vi "Func-엑셀 데이터를 그래프로 출력.vi"() -> ()   [LabVIEW 2015] (continued)
2.46\t3.252\n3.3\t2.47\t3.256\n3.3\t2.48\t3.262\n3.3\t2.49\t3.268\n3.3\t2.5\t3.273\n3.3\t2.51\t3.277\n3.3\t2.51\t3.284\n3.3\t2.52\t3.298\n3.3\t2.52\t3.307\n3.3\t2.52\t3.316\n3.3\t2.53\t3.327\n3.3\t2.54\t3.339\n3.3\t2.55\t3.347\n3.3\t2.56\t3.356\n3.3\t2.57\t3.363\n3.3\t2.57\t3.367\n3.3\t2.58\t3.375\n3.3\t2.59\t3.377\n3.3\t2.6\t3.382\n3.3\t2.6\t3.39\n3.3\t2.61\t3.395\n3.3\t2.61\t3.399\n3.3\t2.62\t3.409\n3.3\t2.63\t3.418\n3.3\t2.63\t3.427\n3.3\t2.64\t3.434\n3.3\t2.65\t3.441\n3.3\t2.66\t3.45\n3.3\t2.66\t3.465\n3.3\t2.67\t3.473\n3.3\t2.68\t3.483\n3.3\t2.68\t3.494\n3.3\t2.69\t3.499\n3.3\t2.69\t3.509\n3.3\t2.69\t3.51\n3.3\t2.7\t3.515\n3.3\t2.71\t3.521\n3.3\t2.72\t3.524\n3.3\t2.72\t3.532\n3.3\t2.73\t3.539\n3.3\t2.73\t3.546\n3.3\t2.74\t3.551\n3.3\t2.74\t3.562\n3.3\t2.75\t3.568\n3.3\t2.75\t3.574\n3.3\t2.76\t3.581\n3.3\t2.77\t3.592\n3.3\t2.78\t3.6\n3.3\t2.78\t3.607\n3.3\t2.78\t3.611\n3.3\t2.79\t3.618\n3.3\t2.79\t3.63\n3.3\t2.8\t3.637\n3.3\t2.81\t3.639\n3.3\t2.81\t3.649\n3.3\t2.82\t3.659\n3.3\t2.83\t3.666\n3.3\t2.83\t3.673\n3.3\t2.84\t3.677\n3.3\t2.84\t3.684\n3.3\t2.85\t3.693\n3.3\t2.86\t3.697\n3.3\t2.86\t3.702\n3.3\t2.86\t3.708\n3.3\t2.86\t3.714\n3.3\t2.87\t3.724\n3.3\t2.87\t3.732\n3.3\t2.88\t3.736\n3.3\t2.89\t3.743\n3.3\t2.9\t3.753\n3.3\t2.9\t3.761\n3.3\t2.91\t3.766\n3.3\t2.91\t3.775\n3.3\t2.92\t3.788\n3.3\t2.92\t3.795\n3.3\t2.93\t3.804\n3.3\t2.93\t3.813\n3.3\t2.94\t3.823\n3.3\t2.94\t3.83\n3.3\t2.94\t3.834\n3.3\t2.95\t3.841\n3.3\t2.95\t3.85\n3.3\t2.96\t3.857\n3.3\t2.96\t3.86\n3.3\t2.97\t3.871\n3.3\t2.97\t3.877\n3.3\t2.98\t3.883\n3.3\t2.98\t3.893\n3.3\t2.99\t3.893\n3.3\t2.99\t3.9\n3.3\t3\t3.911\n3.3\t3\t3.917\n3.3\t3.01\t3.923\n3.3\t3.01\t3.93\n3.3\t3.02\t3.941\n3.3\t3.03\t3.946\n3.3\t3.03\t3.955\n3.3\t3.03\t3.96\n3.3\t3.03\t3.966\n3.3\t3.04\t3.977\n3.3\t3.04\t3.982\n3.3\t3.05\t3.99\n3.3\t3.05\t3.994\n3.3\t3.06\t4.004\n3.3\t3.06\t4.013\n3.3\t3.07\t4.021\n3.3\t3.07\t4.027\n3.3\t3.08\t4.036\n3.3\t3.08\t4.048\n3.3\t3.08\t4.053\n3.3\t3.09\t4.055\n3.3\t3.09\t4.064\n3.3\t3.1\t4.072\n3.3\t3.1\t4.076\n3.3\t3.11\t4.085\n3.3\t3.11\t4.09\n3.3\t3.11\t4.101\n3.3\t3.11\t4.107\n3.3\t3.11\t4.112\n3.3\t3.11\t4.122\n3.3\t3.12\t4.13\n3.3\t3.13\t4.139\n3.3\t3.13\t4.146\n3.3\t3.13\t4.16\n3.3\t3.13\t4.169\n3.3\t3.14\t4.169\n3.3\t3.14\t4.18\n3.3\t3.14\t4.187\n3.3\t3.15\t4.194\n3.3\t3.15\t4.197\n3.3\t3.16\t4.204\n3.3\t3.16\t4.214\n3.3\t3.16\t4.223\n3.3\t3.17\t4.23\n3.3\t3.17\t4.24\n3.3\t3.18\t4.248\n3.3\t3.18\t4.254\n3.3\t3.19\t4.258\n3.3\t3.19\t4.264\n3.3\t3.2\t4.266\n3.3\t3.2\t4.275\n3.3\t3.2\t4.28\n3.3\t3.2\t4.286\n3.3\t3.2\t4.298\n3.3\t3.21\t4.309\n3.3\t3.21\t4.317\n3.3\t3.21\t4.324\n3.3\t3.21\t4.329\n3.3\t3.22\t4.336\n3.3\t3.22\t4.342\n3.3\t3.22\t4.346\n3.3\t3.23\t4.354\n3.3\t3.23\t4.366\n3.3\t3.23\t4.375\n3.3\t3.24\t4.381\n3.3\t3.25\t4.391\n3.3\t3.25\t4.398\n3.3\t3.25\t4.406\n3.3\t3.26\t4.41\n3.3\t3.26\t4.415\n3.3\t3.26\t4.424\n3.3\t3.26\t4.436\n3.3\t3.26\t4.44\n3.3\t3.27\t4.445\n3.3\t3.27\t4.453\n3.3\t3.27\t4.461\n3.3\t3.28\t4.468\n3.3\t3.28\t4.476\n3.3\t3.28\t4.484\n3.3\t3.28\t4.489\n3.3\t3.28\t4.502\n3.3\t3.28\t4.507\n3.3\t3.29\t4.512\n3.3\t3.29\t4.519\n3.3\t3.3\t4.527\n3.3\t3.3\t4.533\n3.3\t3.3\t4.542\n3.3\t3.3\t4.55\n3.3\t3.3\t4.555\n3.3\t3.31\t4.562\n3.3\t3.31\t4.566\n3.3\t3.31\t4.575\n3.3\t3.31\t4.582\n3.3\t3.32\t4.591\n3.3\t3.32\t4.597\n3.3\t3.32\t4.608\n3.3\t3.33\t4.616\n3.3\t3.33\t4.62\n3.3\t3.33\t4.629\n3.3\t3.33\t4.632\n3.3\t3.33\t4.641\n3.3\t3.33\t4.646\n3.3\t3.34\t4.649\n3.3\t3.34\t4.658\n3.3\t3.34\t4.668\n3.3\t3.35\t4.68\n3.3\t3.35\t4.686\n3.3\t3.35\t4.7\n3.3\t3.35\t4.709\n3.3\t3.35\t4.714\n3.3\t3.35\t4.721\n3.3\t3.36\t4.727\n3.3\t3.36\t4.732\n3.3\t3.36\t4.739\n3.3\t3.37\t4.746\n3.3\t3.37\t4.753\n3.3\t3.37\t4.764\n3.3\t3.37\t4.769\n3.3\t3.37\t4.774\n3.3\t3.37\t4.78\n3.3\t3.37\t4.786\n3.3\t3.37\t4.791\n3.3\t3.37\t4.8\n3.3\t3.37\t4.805\n3.3\t3.37\t4.813\n3.3\t3.37\t4.82\n3.3\t3.38\t4.827\n3.3\t3.38\t4.836\n3.3\t3.38\t4.843\n3.3\t3.39\t4.846\n3.3\t3.39\t4.853\n3.3\t3.39\t4.863\n3.3\t3.39\t4.873\n3.3\t3.38\t4.88\n3.3\t3.39\t4.887\n3.3\t3.39\t4.898\n3.3\t3.39\t4.902\n3.3\t3.4\t4.912\n3.3\t3.4\t4.915\n3.3\t3.4\t4.919\n3.3\t3.4\t4.929\n3.3\t3.41\t4.936\n3.3\t3.41\t4.945\n3.3\t3.41\t4.953\n3.3\t3.41\t4.96\n3.3\t3.41\t4.966\n3.3\t3.41\t4.976\n3.3\t3.41\t4.98\n3.3\t3.41\t4.984\n3.3\t3.41\t4.991\n3.3\t3.41\t4.996\n3.3\t3.42\t5.005\n3.3\t3.41\t5.016\n3.3\t3.4\t5.02\n3.3\t3.39\t5.027\n3.3\t3.38\t5.039\n3.3\t3.37\t5.047\n3.3\t3.36\t5.052\n3.3\t3.35\t5.058\n3.3\t3.34\t5.068\n3.3\t3.33\t5.078\n3.3\t3.32\t5.085\n3.3\t3.31\t5.091\n3.3\t3.3\t5.096\n3.3\t3.33\t5.103\n3.3\t3.33\t5.109\n3.3\t3.33\t5.115\n3.3\t3.33\t5.127\n3.3\t3.33\t5.135\n3.3\t3.33\t5.145\n3.3\t3.33\t5.152\n3.3\t3.33\t5.162\n3.3\t3.33\t5.167\n3.3\t3.33\t5.174\n3.3\t3.33\t5.179\n3.3\t3.33\t5.183\n3.3\t3.33\t5.193\n3.3\t3.33\t5.2\n3.3\t3.33\t5.207\n3.3\t3.33\t5.214\n3.3\t3.33\t5.217\n3.3\t3.33\t5.229\n3.3\t3.33\t5.236\n3.3\t3.33\t5.238\n3.3\t3.33\t5.247\n3.3\t3.33\t5.259\n3.3\t3.33\t5.268\n3.3\t3.33\t5.275\n3.3\t3.33\t5.282\n3.3\t3.33\t5.289\n3.3\t3.33\t5.295\n3.3\t3.33\t5.3\n3.3\t3.33\t5.305\n3.3\t3.33\t5.311\n3.3\t3.33\t5.321\n3.3\t3.33\t5.329\n3.3\t3.33\t5.339\n3.3\t3.33\t5.343\n3.3\t3.33\t5.353\n3.3\t3.33\t5.363\n3.3\t3.33\t5.368\n3.3\t3.33\t5.375\n3.3\t3.33\t5.382\n3.3\t3.33\t5.388\n3.3\t3.33\t5.391\n3.3\t3.33\t5.396\n3.3\t3.33\t5.407\n3.3\t3.33\t5.409\n3.3\t3.33\t5.418\n3.3\t3.33\t5.426\n3.3\t3.33\t5.436\n3.3\t3.33\t5.441\n3.3\t3.33\t5.447\n3.3\t3.33\t5.455\n3.3\t3.33\t5.459\n3.3\t3.33\t5.467\n3.3\t3.33\t5.469\n3.3\t3.33\t5.478\n3.3\t3.33\t5.487\n3.3\t3.33\t5.495\n3.3\t3.33\t5.5\n3.3\t3.33\t5.507\n3.3\t3.33\t5.516\n3.3\t3.33\t5.525\n3.3\t3.33\t5.531\n3.3\t3.33\t5.536\n3.3\t3.33\t5.547\n3.3\t3.33\t5.553\n3.3\t3.33\t5.557\n3.3\t3.33\t5.561\n3.3\t3.33\t5.568\n3.3\t3.33\t5.574\n3.3\t3.33\t5.58\n3.3\t3.33\t5.589\n3.3\t3.33\t5.596\n3.3\t3.33\t5.605\n3.3\t3.33\t5.609\n3.3\t3.33\t5.617\n3.3\t3.33\t5.629\n3.3\t3.33\t5.634\n3.3\t3.33\t5.642\n3.3\t3.33\t5.654\n3.3\t3.33\t5.661\n3.3\t3.33\t5.666\n3.3\t3.33\t5.672\n3.3\t3.33\t5.678\n3.3\t3.33\t5.684\n3.3\t3.33\t5.692\n3.3\t3.33\t5.696\n3.3\t3.33\t5.704\n3.3\t3.33\t5.711\n3.3\t3.33\t5.721\n3.3\t3.33\t5.725\n3.3\t3.33\t5.737\n3.3\t3.33\t5.745\n3.3\t3.33\t5.752\n3.3\t3.33\t5.758\n3.3\t3.33\t5.761\n3.3\t3.33\t5.767\n3.3\t3.33\t5.776\n3.3\t3.33\t5.782\n3.3\t3.33\t5.789\n3.3\t3.33\t5.802\n3.3\t3.33\t5.809\n3.3\t3.33\t5.816\n3.3\t3.33\t5.816\n3.3\t3.33\t5.822\n3.3\t3.33\t5.826\n3.3\t3.33\t5.832\n3.3\t3.33\t5.839\n3.3\t3.33\t5.843\n3.3\t3.33\t5.859\n3.3\t3.33\t5.866\n3.3\t3.33\t5.873\n3.3\t3.33\t5.885\n3.3\t3.33\t5.89\n3.3\t3.33\t5.9\n3.3\t3.33\t5.907\n3.3\t3.33\t5.913\n3.3\t3.33\t5.916\n3.3\t3.33\t5.923\n3.3\t3.33\t5.927\n3.3\t3.33\t5.932\n3.3\t3.33\t5.939\n3.3\t3.33\t5.945\n3.3\t3.33\t5.953\n3.3\t3.33\t5.963\n3.3\t3.33\t5.971\n3.3\t3.33\t5.975\n3.3\t3.33\t5.984\n3.3\t3.33\t5.991\n3.3\t3.33\t5.998\n3.3\t3.33\t6.007\n3.3\t3.33\t6.012\n3.3\t3.33\t6.02\n3.3\t3.33\t6.026\n3.3\t3.33\t6.029\n3.3\t3.33\t6.036\n3.3\t3.33\t6.038\n3.3\t3.33\t6.046\n3.3\t3.33\t6.052\n3.3\t3.33\t6.063\n3.3\t3.33\t6.07\n3.3\t3.33\t6.076\n3.3\t3.33\t6.084\n3.3\t3.33\t6.087\n3.3\t3.33\t6.092\n3.3\t3.33\t6.099\n3.3\t3.33\t6.104\n3.3\t3.33\t6.108\n3.3\t3.33\t6.118\n3.3\t3.33\t6.128\n3.3\t3.33\t6.137\n3.3\t3.33\t6.144\n3.3\t3.33\t6.153\n3.3\t3.33\t6.161\n3.3\t3.33\t6.169\n3.3\t3.33\t6.175\n3.3\t3.33\t6.18\n3.3\t3.33\t6.187\n3.3\t3.33\t6.189\n3.3\t3.33\t6.195\n3.3\t3.33\t6.203\n3.3\t3.33\t6.207\n3.3\t3.33\t6.213\n3.3\t3.33\t6.222\n3.3\t3.33\t6.229\n3.3\t3.33\t6.239\n3.3\t3.33\t6.242\n3.3\t3.33\t6.248\n3.3\t3.33\t6.258\n3.3\t3.33\t6.264\n3.3\t3.33\t6.27\n3.3\t3.33\t6.277\n3.3\t3.33\t6.286\n3.3\t3.33\t6.288\n3.3\t3.33\t6.289\n3.3\t3.33\t6.297\n3.3\t3.33\t6.303\n3.3\t3.33\t6.311\n3.3\t3.33\t6.318\n3.3\t3.33\t6.327\n3.3\t3.33\t6.34\n3.3\t3.33\t6.342\n3.3\t3.33\t6.348\n3.3\t3.33\t6.356\n3.3\t3.33\t6.363\n3.3\t3.33\t6.37\n3.3\t3.33\t6.374\n3.3\t3.33\t6.382\n3.3\t3.33\t6.388\n3.3\t3.33\t6.392\n3.3\t3.33\t6.394\n3.3\t3.33\t6.401\n3.3\t3.33\t6.407\n3.3\t3.33\t6.412\n3.3\t3.33\t6.42\n3.3\t3.33\t6.431\n3.3\t3.33\t6.439\n3.3\t3.33\t6.445\n3.3\t3.33\t6.452\n3.3\t3.33\t6.456\n3.3\t3.33\t6.463\n3.3\t3.33\t6.47\n3.3\t3.33\t6.475\n3.3\t3.33\t6.48\n3.3\t3.33\t6.491\n3.3\t3.33\t6.497\n3.3\t3.33\t6.499\n3.3\t3.33\t6.509\n3.3\t3.33\t6.512\n3.3\t3.33\t6.518\n3.3\t3.33\t6.527\n3.3\t3.33\t6.534\n3.3\t3.33\t6.544\n3.3\t3.33\t6.548\n3.3\t3.33\t6.555\n3.3\t3.33\t6.563\n3.3\t3.33\t6.57\n3.3\t3.33\t6.572\n3.3\t3.33\t6.577\n3.3\t3.33\t6.586\n3.3\t3.33\t6.591\n3.3\t3.33\t6.597\n3.3\t3.33\t6.607\n3.3\t3.33\t6.616\n3.3\t3.33\t6.622\n3.3\t3.33\t6.632\n3.3\t3.32\t6.638\n3.3\t3.32\t6.638\n3.3\t3.32\t6.643\n3.3\t3.32\t6.646\n3.3\t3.32\t6.65\n3.3\t3.32\t6.656\n3.3\t3.32\t6.66\n3.3\t3.32\t6.668\n3.3\t3.32\t6.675\n3.3\t3.32\t6.682\n3.3\t3.32\t6.69\n3.3\t3.32\t6.699\n3.3\t3.32\t6.706\n3.3\t3.32\t6.709\n3.3\t3.32\t6.718\n3.3\t3.32\t6.723\n3.3\t3.32\t6.728\n3.3\t3.32\t6.738\n3.3\t3.32\t6.747\n3.3\t3.32\t6.756\n3.3\t3.32\t6.765\n3.3\t3.32\t6.773\n3.3\t3.32\t6.778\n3.3\t3.32\t6.781\n3.3\t3.32\t6.784\n3.3\t3.32\t6.786\n3.3\t3.32\t6.793\n3.3\t3.32\t6.797\n3.3\t3.32\t6.802\n3.3\t3.32\t6.807\n3.3\t3.32\t6.812\n3.3\t3.32\t6.821\n3.3\t3.32\t6.832\n3.3\t3.32\t6.837\n3.3\t3.32\t6.846\n3.3\t3.32\t6.857\n3.3\t3.32\t6.861\n3.3\t3.32\t6.866\n3.3\t3.32\t6.875\n3.3\t3.32\t6.88\n3.3\t3.32\t6.886\n3.3\t3.32\t6.893\n3.3\t3.32\t6.898\n3.3\t3.32\t6.905\n3.3\t3.32\t6.906\n3.3\t3.32\t6.913\n3.3\t3.32\t6.915\n3.3\t3.32\t6.92\n3.3\t3.32\t6.929\n3.3\t3.32\t6.933\n3.3\t3.32\t6.938\n3.3\t3.32\t6.94\n3.3\t3.32\t6.95\n3.3\t3.32\t6.959\n3.3\t3.32\t6.965\n3.3\t3.32\t6.971\n3.3\t3.32\t6.982\n3.3\t3.32\t6.992\n3.3\t3.32\t6.996\n3.3\t3.32\t7.008\n3.3\t3.31\t7.012\n3.3\t3.31\t7.018\n3.3\t3.31\t7.028\n3.3\t3.31\t7.03\n3.3\t3.31\t7.034\n3.3\t3.31\t7.037\n3.3\t3.31\t7.043\n3.3\t3.31\t7.048\n3.3\t3.31\t7.054\n3.3\t3.31\t7.061\n3.3\t3.31\t7.069\n3.3\t3.31\t7.077\n3.3\t3.31\t7.082\n3.3\t3.31\t7.088\n3.3\t3.31\t7.095\n3.3\t3.31\t7.099\n3.3\t3.31\t7.103\n3.3\t3.31\t7.109\n3.3\t3.31\t7.115\n3.3\t3.31\t7.119\n3.3\t3.31\t7.125\n3.3\t3.31\t7.131\n3.3\t3.31\t7.138\n3.3\t3.31\t7.148\n3.3\t3.31\t7.149\n3.3\t3.31\t7.158\n3.3\t3.31\t7.161\n3.3\t3.31\t7.166\n3.3\t3.31\t7.173\n3.3\t3.31\t7.177\n3.3\t3.31\t7.185\n3.3\t3.31\t7.193\n3.3\t3.31\t7.198\n3.3\t3.31\t7.202\n3.3\t3.31\t7.204\n3.3\t3.31\t7.21\n3.3\t3.31\t7.216\n3.3\t3.31\t7.22\n3.3\t3.31\t7.227\n3.3\t3.31\t7.234\n3.3\t3.31\t7.245\n3.3\t3.31\t7.25\n3.3\t3.31\t7.256\n3.3\t3.31\t7.264\n3.3\t3.31\t7.27\n3.3\t3.31\t7.273\n3.3\t3.31\t7.277\n3.3\t3.31\t7.283\n3.3\t3.31\t7.287\n3.3\t3.31\t7.293\n3.3\t3.31\t7.297\n3.3\t3.31\t7.303\n3.3\t3.31\t7.312\n3.3\t3.31\t7.317\n3.3\t3.31\t7.325\n3.3\t3.31\t7.336\n3.3\t3.31\t7.343\n3.3\t3.31\t7.349\n3.3\t3.31\t7.354\n3.3\t3.31\t7.358\n3.3\t3.31\t7.358\n3.3\t3.31\t7.362\n3.3\t3.31\t7.37\n3.3\t3.31\t7.372\n3.3\t3.31\t7.377\n3.3\t3.31\t7.383\n3.3\t3.31\t7.393\n3.3\t3.31\t7.4\n3.3\t3.31\t7.401\n3.3\t3.31\t7.41\n3.3\t3.31\t7.423\n3.3\t3.31\t7.426\n3.3\t3.31\t7.43\n3.3\t3.31\t7.434\n3.3\t3.31\t7.443\n3.3\t3.31\t7.447\n3.3\t3.31\t7.452\n3.3\t3.31\t7.458\n3.3\t3.31\t7.463\n3.3\t3.3\t7.475\n3.3\t3.31\t7.476\n3.3\t3.31\t7.48\n3.3\t3.31\t7.485\n3.3\t3.31\t7.493\n3.3\t3.31\t7.497\n3.3\t3.31\t7.503\n3.3\t3.31\t7.511\n3.3\t3.31\t7.517\n3.3\t3.31\t7.529\n3.3\t3.31\t7.534\n3.3\t3.3\t7.537\n3.3\t3.3\t7.545\n3.3\t3.3\t7.549\n3.3\t3.3\t7.553\n3.3\t3.3\t7.557\n3.3\t3.3\t7.561\n3.3\t3.3\t7.569\n3.3\t3.3\t7.579\n3.3\t3.3\t7.582\n3.3\t3.3\t7.587\n3.3\t3.3\t7.592\n3.3\t3.3\t7.597\n3.3\t3.3\t7.604\n3.3\t3.3\t7.607\n3.3\t3.3\t7.611\n3.3\t3.31\t7.616\n3.3\t3.31\t7.621\n3.3\t3.31\t7.627\n3.3\t3.31\t7.625\n3.3\t3.31\t7.63\n3.3\t3.31\t7.636\n3.3\t3.31\t7.639\n3.3\t3.31\t7.648\n3.3\t3.31\t7.648\n3.3\t3.31\t7.658\n3.3\t3.31\t7.665\n3.3\t3.31\t7.67\n3.3\t3.31\t7.678\n3.3\t3.31\t7.687\n3.3\t3.31\t7.694\n3.3\t3.31\t7.693\n3.3\t3.31\t7.702\n3.3\t3.31\t7.706\n3.3\t3.31\t7.711\n3.3\t3.31\t7.714\n3.3\t3.31\t7.72\n3.3\t3.31\t7.728\n3.3\t3.31\t7.73\n3.3\t3.31\t7.739\n3.3\t3.31\t7.742\n3.3\t3.31\t7.748\n3.3\t3.31\t7.752\n3.3\t3.31\t7.758\n3.3\t3.31\t7.767\n3.3\t3.31\t7.769\n3.3\t3.31\t7.776\n3.3\t3.31\t7.782\n3.3\t3.31\t7.789\n3.3\t3.31\t7.793\n3.3\t3.31\t7.796\n3.3\t3.31\t7.801\n3.3\t3.31\t7.807\n3.3\t3.31\t7.81\n3.3\t3.31\t7.815\n3.3\t3.31\t7.818\n3.3\t3.31\t7.827\n3.3\t3.31\t7.832\n3.3\t3.31\t7.836\n3.3\t3.31\t7.843\n3.3\t3.31\t7.847\n3.3\t3.31\t7.853\n3.3\t3.31\t7.86\n3.3\t3.3\t7.866\n3.3\t3.3\t7.871\n3.3\t3.3\t7.879\n3.3\t3.31\t7.885\n3.3\t3.31\t7.892\n3.3\t3.31\t7.898\n3.3\t3.31\t7.905\n3.3\t3.31\t7.911\n3.3\t3.31\t7.913\n3.3\t3.3\t7.917\n3.3\t3.3\t7.921\n3.3\t3.3\t7.928\n3.3\t3.3\t7.929\n3.3\t3.3\t7.93\n3.3\t3.3\t7.938\n3.3\t3.3\t7.941\n3.3\t3.3\t7.948\n3.3\t3.3\t7.952\n3.3\t3.3\t7.959\n3.3\t3.3\t7.971\n3.3\t3.3\t7.976\n3.3\t3.3\t7.982\n3.3\t3.3\t7.984\n3.3\t3.3\t7.987\n3.3\t3.3\t7.988\n3.3\t3.3\t7.993\n3.3\t3.3\t7.995\n3.3\t3.3\t8\n3.3\t3.3\t8.008\n3.3\t3.3\t8.014\n3.3\t3.3\t8.018\n3.3\t3.3\t8.023\n3.3\t3.3\t8.026\n3.3\t3.3\t8.026\n3.3\t3.3\t8.033\n3.3\t3.3\t8.036\n3.3\t3.3\t8.043\n3.3\t3.3\t8.049\n3.3\t3.3\t8.055\n3.3\t3.3\t8.064\n3.3\t3.3\t8.066\n3.3\t3.3\t8.073\n3.3\t3.3\t8.079\n3.3\t3.3\t8.087\n3.3\t3.3\t8.094\n3.3\t3.3\t8.099\n3.3\t3.3\t8.108\n3.3\t3.3\t8.111\n3.3\t3.3\t8.112\n3.3\t3.3\t8.117\n3.3\t3.3\t8.122\n3.3\t3.3\t8.123\n3.3\t3.3\t8.128\n3.3\t3.3\t8.13\n3.3\t3.3\t8.137\n3.3\t3.3\t8.141\n3.3\t3.3\t8.141\n3.3\t3.3\t8.148\n3.3\t3.3\t8.157\n3.3\t3.3\t8.162\n3.3\t3.3\t8.168\n3.3\t3.3\t8.177\n3.3\t3.3\t8.185\n3.3\t3.3\t8.19\n3.3\t3.3\t8.192\n3.3\t3.3\t8.195\n3.3\t3.3\t8.203\n3.3\t3.3\t8.208\n3.3\t3.3\t8.211\n3.3\t3.3\t8.22\n3.3\t3.3\t8.222\n3.3\t3.3\t8.232\n3.3\t3.3\t8.236\n3.3\t3.3\t8.238\n3.3\t3.3\t8.242\n3.3\t3.3\t8.248\n3.3\t3.3\t8.253\n3.3\t3.3\t8.254\n3.3\t3.3\t8.261\n3.3\t3.3\t8.265\n3.3\t3.3\t8.272\n3.3\t3.3\t8.276\n3.3\t3.3\t8.281\n3.3\t3.3\t8.287\n3.3\t3.3\t8.292\n3.3\t3.3\t8.297\n3.3\t3.3\t8.3\n3.3\t3.3\t8.305\n3.3\t3.3\t8.31\n3.3\t3.3\t8.315\n3.3\t3.3\t8.322\n3.3\t3.3\t8.326\n3.3\t3.3\t8.331\n3.3\t3.3\t8.336\n3.3\t3.3\t8.343\n3.3\t3.3\t8.346\n3.3\t3.3\t8.35\n3.3\t3.3\t8.353\n3.3\t3.3\t8.355\n3.3\t3.3\t8.364\n3.3\t3.3\t8.364\n3.3\t3.3\t8.367\n3.3\t3.3\t8.377\n3.3\t3.3\t8.384\n3.3\t3.3\t8.393\n3.3\t3.3\t8.393\n3.3\t3.3\t8.396\n3.3\t3.3\t8.4\n3.3\t3.3\t8.403\n3.3\t3.3\t8.406\n3.3\t3.3\t8.407\n3.3\t3.3\t8.413\n3.3\t3.3\t8.422\n3.3\t3.3\t8.428\n3.3\t3.3\t8.43\n3.3\t3.3\t8.434\n3.3\t3.3\t8.442\n3.3\t3.3\t8.447\n3.3\t3.3\t8.45\n3.3\t3.3\t8.454\n3.3\t3.3\t8.457\n3.3\t3.3\t8.464\n3.3\t3.3\t8.473\n3.3\t3.3\t8.475\n3.3\t3.3\t8.479\n3.3\t3.3\t8.484\n3.3\t3.3\t8.488\n3.3\t3.3\t8.489\n3.3\t3.3\t8.489\n3.3\t3.3\t8.491\n3.3\t3.3\t8.496\n3.3\t3.3\t8.504\n3.3\t3.3\t8.509\n3.3\t3.3\t8.513\n3.3\t3.3\t8.523\n3.3\t3.3\t8.529\n3.3\t3.3\t8.531\n3.3\t3.3\t8.533\n3.3\t3.3\t8.538\n3.3\t3.3\t8.54\n3.3\t3.3\t8.546\n3.3\t3.3\t8.548\n3.3\t3.3\t8.554\n3.3\t3.3\t8.562\n3.3\t3.3\t8.568\n3.3\t3.3\t8.575\n3.3\t3.3\t8.579\n3.3\t3.3\t8.584\n3.3\t3.3\t8.592\n3.3\t3.3\t8.596\n3.3\t3.3\t8.601\n3.3\t3.3\t8.603\n3.3\t3.3\t8.607\n3.3\t3.3\t8.613\n3.3\t3.3\t8.611\n3.3\t3.3\t8.617\n3.3\t3.3\t8.62\n3.3\t3.3\t8.625\n3.3\t3.3\t8.63\n3.3\t3.3\t8.632\n3.3\t3.3\t8.637\n3.3\t3.3\t8.643\n3.3\t3.3\t8.645\n3.3\t3.3\t8.651\n3.3\t3.3\t8.656\n3.3\t3.3\t8.661\n3.3\t3.3\t8.667\n3.3\t3.3\t8.672\n3.3\t3.3\t8.676\n3.3\t3.3\t8.681\n3.3\t3.3\t8.684\n3.3\t3.3\t8.688\n3.3\t3.3\t8.691\n3.3\t3.3\t8.695\n3.3\t3.3\t8.698\n3.3\t3.3\t8.705\n3.3\t3.3\t8.711\n3.3\t3.3\t8.714\n3.3\t3.3\t8.721\n3.3\t3.3\t8.726\n3.3\t3.3\t8.729\n3.3\t3.3\t8.733\n3.3\t3.3\t8.738\n3.3\t3.3\t8.739\n3.3\t3.3\t8.739\n3.3\t3.3\t8.745\n3.3\t3.3\t8.75\n3.3\t3.3\t8.754\n3.3\t3.3\t8.758\n3.3\t3.3\t8.766\n3.3\t3.3\t8.777\n3.3\t3.3\t8.779\n3.3\t3.3\t8.78\n3.3\t3.3\t8.785\n3.3\t3.3\t8.786\n3.3\t3.3\t8.792\n3.3\t3.3\t8.797\n3.3\t3.3\t8.8\n3.3\t3.3\t8.809\n3.3\t3.3\t8.817\n3.3\t3.3\t8.824\n3.3\t3.3\t8.824\n3.3\t3.3\t8.828\n3.3\t3.3\t8.834\n3.3\t3.3\t8.836\n3.3\t3.3\t8.841\n3.3\t3.3\t8.848\n3.3\t3.3\t8.853\n3.3\t3.3\t8.856\n3.3\t3.3\t8.858\n3.3\t3.3\t8.856\n3.3\t3.3\t8.863\n3.3\t3.3\t8.861\n3.3\t3.3\t8.863\n3.3\t3.3\t8.87\n3.3\t3.3\t8.873\n3.3\t3.3\t8.881\n3.3\t3.3\t8.885\n3.3\t3.3\t8.889\n3.3\t3.3\t8.895\n3.3\t3.3\t8.896\n3.3\t3.3\t8.904\n3.3\t3.3\t8.908\n3.3\t3.3\t8.911\n3.3\t3.3\t8.916\n3.3\t3.3\t8.92\n3.3\t3.3\t8.925\n3.3\t3.3\t8.928\n3.3\t3.3\t8.935\n3.3\t3.3\t8.941\n3.3\t3.3\t8.942\n3.3\t3.3\t8.944\n3.3\t3.3\t8.95\n3.3\t3.3\t8.953\n3.3\t3.3\t8.956\n3.3\t3.3\t8.959\n3.3\t3.3\t8.966\n3.3\t3.3\t8.97\n3.3\t3.3\t8.973\n3.3\t3.3\t8.98\n3.3\t3.3\t8.986\n3.3\t3.3\t8.989\n3.3\t3.3\t8.992\n3.3\t3.3\t8.999\n3.3\t3.3\t9.003\n3.3\t3.3\t9.005\n3.3\t3.3\t9.006\n3.3\t3.3\t9.014\n3.3\t3.3\t9.018\n3.3\t3.3\t9.025\n3.3\t3.3\t9.025\n3.3\t3.3\t9.028\n3.3\t3.3\t9.032\n3.3\t3.3\t9.035\n3.3\t3.3\t9.037\n3.3\t3.3\t9.043\n3.3\t3.3\t9.049\n3.3\t3.3\t9.052\n3.3\t3.3\t9.06\n3.3\t3.3\t9.062\n3.3\t3.3\t9.07\n3.3\t3.3\t9.072\n3.3\t3.3\t9.074\n3.3\t3.3\t9.077\n3.3\t3.3\t9.082\n3.3\t3.3\t9.085\n3.3\t3.3\t9.082\n3.3\t3.3\t9.089\n3.3\t3.3\t9.095\n3.3\t3.3\t9.101\n3.3\t3.3\t9.103\n3.3\t3.3\t9.105\n3.3\t3.3\t9.112\n3.3\t3.3\t9.115\n3.3\t3.3\t9.118\n3.3\t3.3\t9.116\n3.3\t3.3\t9.123\n3.3\t3.3\t9.129\n3.3\t3.3\t9.13\n3.3\t3.3\t9.134\n3.3\t3.3\t9.14\n3.3\t3.3\t9.148\n3.3\t3.3\t9.151\n3.3\t3.3\t9.151\n3.3\t3.3\t9.156\n3.3\t3.3\t9.16\n3.3\t3.3\t9.159\n3.3\t3.3\t9.161\n3.3\t3.3\t9.165\n3.3\t3.3\t9.172\n3.3\t3.3\t9.18\n3.3\t3.3\t9.186\n3.3\t3.3\t9.193\n3.3\t3.3\t9.198\n3.3\t3.3\t9.201\n3.3\t3.3\t9.202\n3.3\t3.3\t9.204\n3.3\t3.3\t9.206\n3.3\t3.3\t9.208\n3.3\t3.3\t9.212\n3.3\t3.3\t9.214\n3.3\t3.3\t9.218\n3.3\t3.3\t9.226\n3.3\t3.3\t9.229\n3.3\t3.3\t9.232\n3.3\t3.3\t9.237\n3.3\t3.3\t9.238\n3.3\t3.3\t9.239\n3.3\t3.3\t9.239\n3.3\t3.3\t9.242\n3.3\t3.3\t9.246\n3.3\t3.3\t9.251\n3.3\t3.3\t9.259\n3.3\t3.3\t9.268\n3.3\t3.3\t9.276\n3.3\t3.3\t9.279\n3.3\t3.3\t9.284\n3.3\t3.3\t9.285\n3.3\t3.3\t9.287\n3.3\t3.3\t9.288\n3.3\t3.3\t9.289\n3.3\t3.3\t9.295\n3.3\t3.3\t9.295\n3.3\t3.3\t9.304\n3.3\t3.3\t9.306\n3.3\t3.3\t9.307\n3.3\t3.3\t9.312\n3.3\t3.3\t9.313\n3.3\t3.3\t9.316\n3.3\t3.3\t9.321\n3.3\t3.3\t9.325\n3.3\t3.3\t9.33\n3.3\t3.3\t9.338\n3.3\t3.3\t9.337\n3.3\t3.3\t9.341\n3.3\t3.3\t9.342\n3.3\t3.3\t9.346\n3.3\t3.3\t9.351\n3.3\t3.3\t9.35\n3.3\t3.3\t9.359\n3.3\t3.3\t9.365\n3.3\t3.3\t9.371\n3.3\t3.3\t9.375\n3.3\t3.3\t9.378\n3.3\t3.3\t9.384\n3.3\t3.3\t9.384\n3.3\t3.3\t9.385\n3.3\t3.3\t9.39\n3.3\t3.3\t9.391\n3.3\t3.3\t9.392\n3.3\t3.3\t9.393\n3.3\t3.3\t9.4\n3.3\t3.3\t9.402\n3.3\t3.3\t9.404\n3.3\t3.3\t9.409\n3.3\t3.3\t9.414\n3.3\t3.3\t9.418\n3.3\t3.3\t9.416\n3.3\t3.3\t9.423\n3.3\t3.3\t9.423\n3.3\t3.3\t9.427\n3.3\t3.3\t9.43\n3.3\t3.3\t9.436\n3.3\t3.3\t9.441\n3.3\t3.3\t9.44\n3.3\t3.3\t9.448\n3.3\t3.3\t9.451\n3.3\t3.3\t9.454\n3.3\t3.3\t9.455\n3.3\t3.3\t9.463\n3.3\t3.3\t9.466\n3.3\t3.3\t9.47\n3.3\t3.3\t9.472\n3.3\t3.3\t9.477\n3.3\t3.3\t9.479\n3.3\t3.3\t9.479\n3.3\t3.3\t9.486\n3.3\t3.3\t9.487\n3.3\t3.3\t9.489\n3.3\t3.3\t9.491\n3.3\t3.3\t9.494\n3.3\t3.3\t9.494\n3.3\t3.3\t9.497\n3.3\t3.3\t9.5\n3.3\t3.3\t9.505\n3.3\t3.3\t9.511\n3.3\t3.3\t9.512\n3.3\t3.3\t9.518\n3.3\t3.3\t9.521\n3.3\t3.3\t9.525\n3.3\t3.3\t9.529\n3.3\t3.3\t9.533\n3.3\t3.3\t9.538\n3.3\t3.3\t9.539\n3.3\t3.3\t9.548\n3.3\t3.3\t9.55\n3.3\t3.3\t9.553\n3.3\t3.3\t9.557\n3.3\t3.3\t9.561\n3.3\t3.3\t9.565\n3.3\t3.3\t9.568\n3.3\t3.3\t9.571\n3.3\t3.3\t9.57\n3.3\t3.3\t9.576\n3.3\t3.3\t9.577\n3.3\t3.3\t9.578\n3.3\t3.3\t9.583\n3.3\t3.3\t9.583\n3.3\t3.3\t9.586\n3.3\t3.3\t9.584\n3.3\t3.3\t9.589\n3.3\t3.3\t9.594\n3.3\t3.3\t9.596\n3.3\t3.3\t9.603\n3.3\t3.3\t9.609\n3.3\t3.3\t9.616\n3.3\t3.3\t9.618\n3.3\t3.3\t9.62\n3.3\t3.3\t9.624\n3.3\t3.3\t9.627\n3.3\t3.3\t9.628\n3.3\t3.3\t9.636\n3.3\t3.3\t9.636\n3.3\t3.3\t9.637\n3.3\t3.3\t9.644\n3.3\t3.3\t9.644\n3.3\t3.3\t9.647\n3.3\t3.3\t9.643\n3.3\t3.3\t9.647\n3.3\t3.3\t9.652\n3.3\t3.3\t9.655\n3.3\t3.3\t9.659\n3.3\t3.3\t9.667\n3.3\t3.3\t9.671\n3.3\t3.3\t9.674\n3.3\t3.3\t9.675\n3.3\t3.3\t9.675\n3.3\t3.3\t9.675\n3.3\t3.3\t9.675\n3.3\t3.3\t9.68\n3.3\t3.3\t9.684\n3.3\t3.3\t9.691\n3.3\t3.3\t9.693\n3.3\t3.3\t9.693\n3.3\t3.3\t9.697\n3.3\t3.3\t9.7\n3.3\t3.3\t9.702\n3.3\t3.3\t9.703\n3.3\t3.3\t9.705\n3.3\t3.3\t9.714\n3.3\t3.3\t9.714\n3.3\t3.3\t9.717\n3.3\t3.3\t9.721\n3.3\t3.3\t9.729\n3.3\t3.3\t9.734\n3.3\t3.3\t9.734\n3.3\t
